vi "Merge Data.vi"(8 "error in":errorcluster, 10 "Analyzed":refnum<class "Instrument.lvclass">, 11 "Acquired":refnum<class "nPAS.lvclass">) -> (0 "error out":errorcluster, 3 "nPAS out":refnum<class "nPAS.lvclass">)   [LabVIEW 2018, in "gPAS Library.lvlib" / "nPAS.lvclass"]
doc: "Merge the analyzed data with that of the current retrieved data set. In this case, we are only concerned with insuring that the cell quality and resonant frequency are properly populated."
uses:
  nPAS.lvclass
  C:/Program Files (x86)/National Instruments/LabVIEW 2018/vi.lib/MSR Consulting, LLC/General Reuse/Instrument/Instrument.lvclass
  <vilib>/MSR Consulting, LLC/General Reuse/Instrument/Instrument.lvclass
  nPAS.lvclass/nPAS.ctl
  <vilib>/MSR Consulting, LLC/General Reuse/PAS/Data/Main/PAS Data.lvclass
  <vilib>/MSR Consulting, LLC/General Reuse/Instrument/Instrument.lvclass/Instrument.ctl
  <vilib>/MSR Consulting, LLC/General Reuse/PAS/Data/Cell/PAS Cell Data.lvclass
  <vilib>/MSR Consulting, LLC/General Reuse/Instrument/Read Data.vi
  <vilib>/MSR Consulting, LLC/General Reuse/PAS/Data/Main/Read CellData.vi
  <vilib>/MSR Consulting, LLC/General Reuse/PAS/Data/Cell/Read timeData.vi
  <vilib>/MSR Consulting, LLC/General Reuse/PAS/Data/Cell/Read lasDiodeData.vi
  <vilib>/MSR Consulting, LLC/General Reuse/PAS/Main/PAS.lvclass
  <vilib>/MSR Consulting, LLC/General Reuse/Data/Data.lvclass
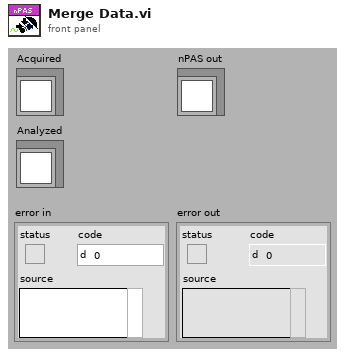
[diagram p1: front panel]
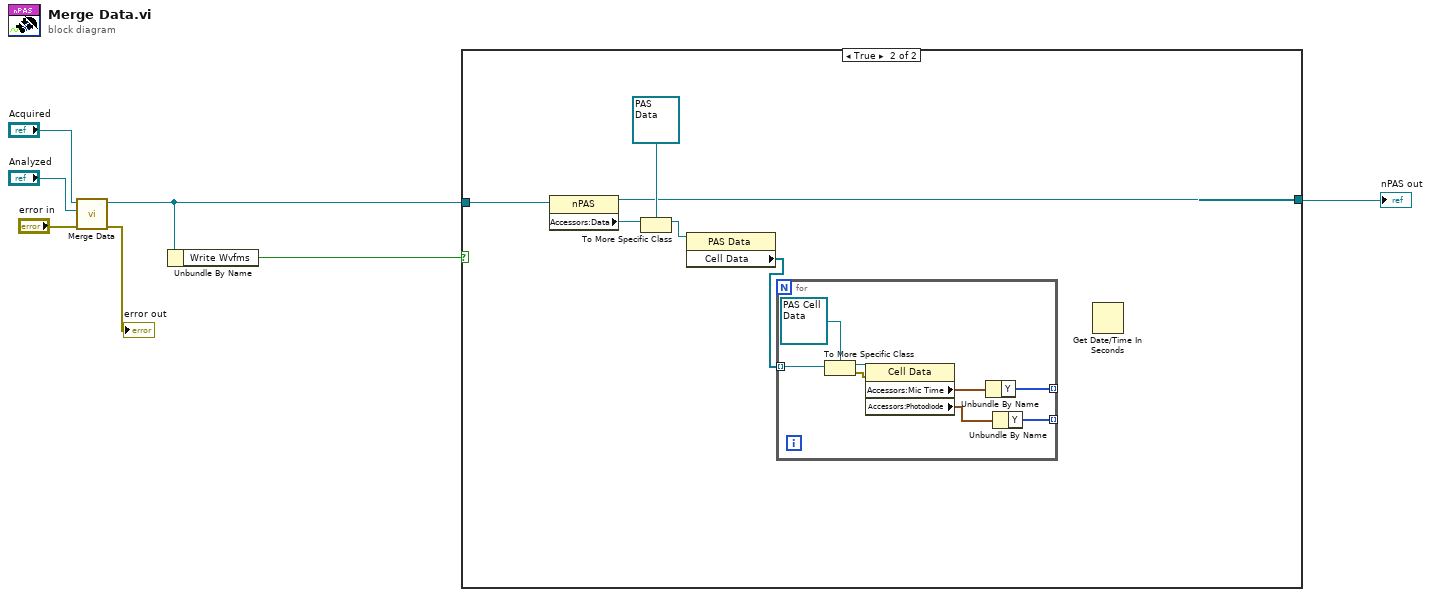
[diagram p0: block diagram]
diagram:
  n1 = call-parent "Merge Data.vi"("error in"="error in", "Analyzed"="Analyzed", "Acquired"="Acquired") -> ("error out"=→"error out":errorcluster, "PAS out"=w2:refnum<class "nPAS.lvclass">)  [unwired: 7 in]
  n2 = Unbundle By Name(w2) -> ("Write Wvfms"=w3:bool)
  n3 = case shown="True" w3 {
    tunnel: w2 -> [w8 w12]
    tunnel: [w8 w11] -> w1
    frame False {
    }
    frame True {
      n4 = property class="nPAS"(reference=w12) -> (reference out=w11:refnum<class "nPAS.lvclass">, "Accessors:Data"=w14:refnum<class "Data.lvclass">)  [unwired: 1 in, 1 out]
      n5 = To More Specific Class(target class=refnum<class "PAS Data.lvclass"> refnum ("PAS Library.lvlib:PAS Data"), reference=w14) -> (specific class reference=w10:refnum<class "PAS Data.lvclass">)  [unwired: 1 in, 1 out]
      n6 = property class="PAS Data"(reference=w10) -> ("Cell Data"=w9:refnum<class "PAS Cell Data.lvclass">[])  [unwired: 1 in, 2 out]
      n7 = for {
        tunnel: w9 -> [w22] mode=indexing
        tunnel: [w17] -> _ mode=indexing
        tunnel: [w15] -> _ mode=indexing
        n8 = To More Specific Class(target class=refnum<class "PAS Cell Data.lvclass"> refnum ("PAS Library.lvlib:Cell Data"), reference=w22) -> (specific class reference=w19:refnum<class "PAS Cell Data.lvclass">, error out=w20:errorcluster)  [unwired: 1 in]
        n9 = property class="Cell Data"(reference=w19, error in=w20) -> ("Accessors:Mic Time"=w18:waveform(i16), "Accessors:Photodiode"=w16:waveform(i16))  [unwired: 2 out]
        n10 = Unbundle By Name(w18) -> ("Y"=w17:i16[])
        n11 = Unbundle By Name(w16) -> ("Y"=w15:i16[])
      }
      n12 = Get Date/Time In Seconds() -> ()  [unwired: 1 out]
    }
  }
  "nPAS out" <- w1
